vi "Nonfunctional Low rep rate beam pointing correction from kHz images.vi"() -> ()   [LabVIEW 2020]
doc: "The Parallel Processing (Optimized Performance) example shows how to process multiple images in parallel when using a ring acquisition. Images acquired from a camera are stored in a ring buffer and references to each image are pushed to a queue. Each worker loop removes a reference from the queue and processes the image.\n\nIn this example, image processing is simulated by a time delay that can be adjusted while the VI is running. When processing is complete, <B>IMAQdx Release Image</B> must be called in order to free space in the ring buffer."
uses:
  <vilib>/vision/Image Controls.llb/IMAQ Image.ctl
  <vilib>/vision/driver/IMAQdx.llb/IMAQdx Acquisition Mode.ctl
  <vilib>/vision/driver/IMAQdx.llb/IMAQdx Buffer Number Mode.ctl
  <vilib>/vision/driver/NI_Vision_Acquisition_Software.lvlib
  <resource>/objmgr/imaqdx.rc
panel:
  out "remaining elements":T2(array[cluster])
  out "# elements in queue":i32
  out "error out":errorcluster
  out "loop time":u32
  out "Waveform Chart":T3(graph)
  out "Image":T1(plugin-control)
  in  "threshold fraction":sgl=0.8
  in  "Use threshold fraction":bool=TRUE
  out "Images Saved Per Second":dbl
  out "Images Acquired Per Second":dbl
  out "Images Behind":u32
  in  "Range":cluster{"Lower value":sgl, "Upper value":sgl}={"Lower value"=128.0, "Upper value"=255.0} caption="Threshold Range" {"Upper value" format="%.2f"; "Lower value" format="%.2f"}
  out "Lost Buffer Count":u32
  in  "Max # images in memory":i32=200
  out "Images in Queue":i32
  out "Images Processed":u32
  out "Current Buffer Number":u32
  in  "Camera Name":refnum<k21> caption="IMAQdx Session"
  in  "Stop":bool
  # "Overview: Processes multiple extracted images in parallel when using a ring acquisition.\nRequirements: Vision Acquisition Software\nInstructions:\n1. Select the Camera Name\n2. Run the VI"
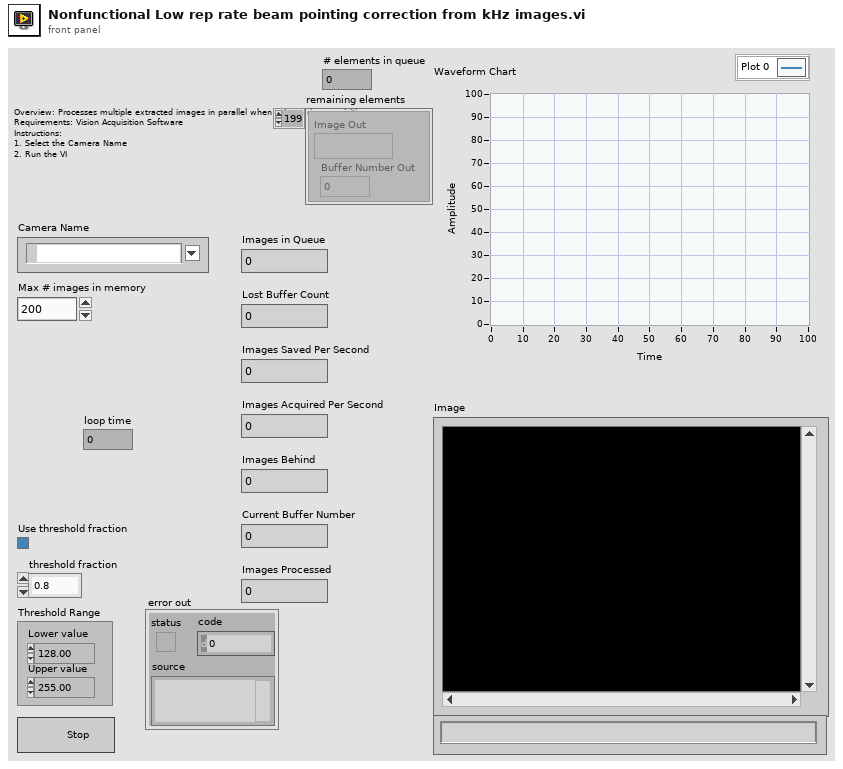
[diagram p1: front panel]
types:
  T1 = typedef "IMAQ Image.ctl" = refnum<image>
  T2 = cluster{"Image Out":T1, "Buffer Number Out":u32}[]
  T3 = cluster{"X Centroid":sgl, "Y Centroid":sgl, "X Centroid":sgl, "Y Centroid":sgl}
  T4 = typedef "IMAQdx.ctl" = refnum<k21>
  T5 = typedef "NI_Vision_Acquisition_Software.lvlib/IMAQdx Acquisition Mode.ctl" = enum32{"One Shot", "Continuous"}
  T6 = typedef "NI_Vision_Acquisition_Software.lvlib/IMAQdx Buffer Number Mode.ctl" = enum32{"Next", "Last", "Buffer Number", "Every", "Last New"}
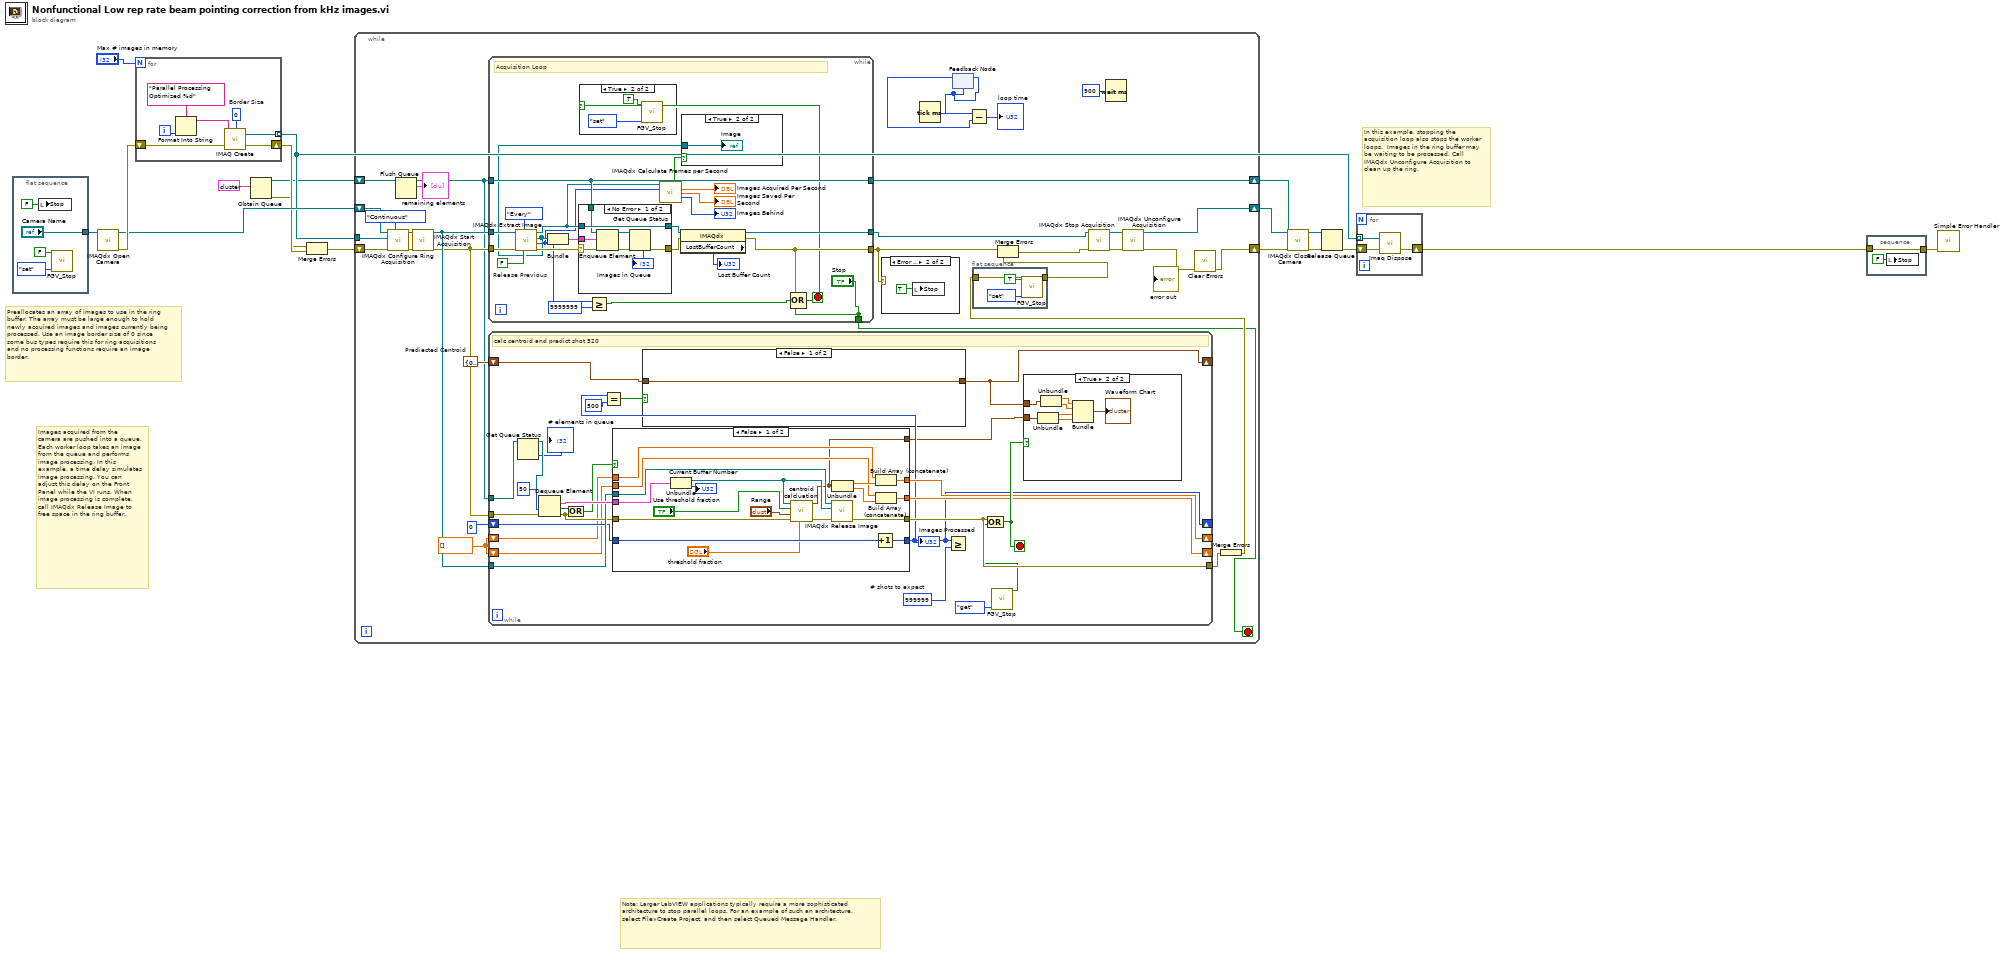
[diagram p0: block diagram]
diagram:
  # "In this example, stopping the acquisition loop also stops the worker loops.  Images in the ring buffer may be waiting to be processed. Call IMAQdx Unconfigure Acquisition to clean up the ring."
  # "Images acquired from the camera are pushed into a queue. Each worker loop takes an image from the queue and performs image processing. In this example, a time delay simulates image processing. You can adjust this delay on the Front Panel while the VI runs. When image processing is complete, call IMAQdx Release Image to free space in the ring buffer."
  # "Preallocates an array of images to use in the ring buffer. The array must be large enough to hold newly acquired images and images currently being processed. Use an image border size of 0 since some bus types require this for ring acquisitions and no processing functions require an image border."
  # "Note: Larger LabVIEW applications typically require a more sophisticated architecture to stop parallel loops. For an example of such an architecture, select File»Create Project, and then select Queued Message Handler."
  n1 = flat-sequence {
    tunnel: ["Camera Name"] -> w15
    frame #0 {
      n2 = local write "Stop"(FALSE ("Stop")) -> ()
      n3 = call "FGV_Stop.vi"("command"=enum16{"set", "get"}."set", "stop"=FALSE) -> ()  [unwired: 9 in, 1 out]
    }
  }
  n4 = call <vilib>:"IMAQdx Open Camera.vi"("Session In"=w15) -> ("error out"=w12:errorcluster, "Session Out"=w11:T4)  [unwired: 2 in, 7 out]
  n5 = for {
    N: "Max # images in memory" -> [_]
    tunnel: [w27] -> w4 mode=indexing
    shift-right: [w26] -> w8
    shift-left: w12 -> [w28]
    i -> [w25]
    w22 = 0  # Border Size
    n6 = Format Into String(format string="Parallel Processing Optimized %d" ("Image Name"), w25) -> (resulting string=w24:string)  [unwired: 2 in, 1 out]
    n7 = call "IMAQ Create"("Border Size"=w22, "Image Name"=w24, "error in (no error)"=w28) -> ("New Image"=w27:T1, "error out"=w26:errorcluster)  [unwired: 1 in, 1 out]
  }
  n8 = Obtain Queue(element data type=cluster{"Image Out":T1, "Buffer Number Out":u32} {"Image Out"=refnum, "Buffer Number Out"=0}) -> (queue out=w1:refnum<queue>, error out=w7:errorcluster)  [unwired: 4 in, 1 out]
  n9 = Merge Errors(w7, w8) -> (w9:errorcluster)
  n10 = while {
    tunnel: w4 -> [w49]
    shift-right: [w59] -> w13
    shift-left: w11 -> [w54]
    shift-right: [w34] -> w14
    shift-left: w9 -> [w52]
    shift-right: [w50] -> w5
    shift-left: w1 -> [w32]
    stop <- w29 stop-if-true
    w39 = cluster{"X Centroid":sgl, "Y Centroid":sgl} {"X Centroid"=0.0, "Y Centroid"=0.0}  # Prediected Centroid
    w40 = sgl[] []
    n11 = call <vilib>:"IMAQdx Configure Ring Acquisition.vi"("Mode"=IMAQdx_Acquisition_Mode."Continuous" ("Continuous?"), "error in"=w52, "Images"=w49, "Session In"=w54) -> ("error out"=w55:errorcluster, "Session Out"=w56:T4)  [unwired: 5 in, 1 out]
    n12 = Flush Queue(queue=w32) -> (queue out=w31:refnum<queue>, remaining elements=→"remaining elements":T2)  [unwired: 1 in, 1 out]
    n13 = call <vilib>:"IMAQdx Start Acquisition.vi"("error in"=w55, "Session In"=w56) -> ("error out"=w46:errorcluster, "Session Out"=w47:T4)  [unwired: 8 out]
    n14 = while {
      tunnel: w46 -> [w144]
      tunnel: w47 -> [w141]
      tunnel: w31 -> [w134]
      tunnel: [w140] -> w48
      tunnel: [w138] -> w45
      tunnel: [w134] -> w50
      tunnel: ["Stop"] -> w29
      stop <- w122 stop-if-true
      w142 = FALSE  # Release Previous
      # "Acquisition Loop"
      n15 = call <vilib>:"IMAQdx Extract Image.vi"("Release Previous (true)"=w142, "Buffer Number Mode (Next)"=IMAQdx_Buffer_Number_Mode."Every" ("Buffer Number Mode"), "error in"=w144, "Session In"=w141) -> ("error out"=w137:errorcluster, "Buffer Number Out"=w125:u32, "Image Out"=w127:T1, "Session Out"=w129:T4)  [unwired: 4 in]
      n16 = Bundle("Image Out"=w127, "Buffer Number Out"=w125) -> (w135:cluster{"Image Out":T1, "Buffer Number Out":u32})  [unwired: 1 in]
      n17 = case shown="No Error" w137 {
        selector: w137 -> [w151 w156]
        tunnel: [w152 w157] -> w136
        tunnel: w129 -> [w152 w157]
        tunnel: w135 -> [w150 _]
        tunnel: w134 -> [w149 _]
        tunnel: [w148 w156] -> w133
        frame No Error {
          n18 = Enqueue Element(queue=w149, element=w150, error in (no error)=w151) -> (queue out=w154:refnum<queue>, error out=w155:errorcluster)  [unwired: 1 in, 1 out]
          n19 = Get Queue Status(queue=w154, error in (no error)=w155) -> (error out=w148:errorcluster, # elements in queue=→"Images in Queue":i32)  [unwired: 1 in, 6 out]
        }
        frame Error {
        }
      }
      n20 = Greater Or Equal?(x=w125, y=u32 9999999) -> (x >= y?=w123:bool)
      n21 = call <vilib>:"IMAQdx Calculate Frames per Second.vi"("Session In"=w129, "Buffer Number"=w125) -> ("Update Display"=w128:bool, "Acquired Frames per Second"=→"Images Acquired Per Second":dbl, "Processed Frames per Second"=→"Images Saved Per Second":dbl, "Images Behind"=→"Images Behind":i32)  [unwired: 7 in, 3 out]
      n22 = property class="IMAQdx"(reference=w136, error in=w133) -> (reference out=w140:T4, error out=w138:errorcluster, "LostBufferCount"=→"Lost Buffer Count":u32)
      n23 = case shown="True" w128 {
        tunnel: w127 -> [_ w147]
        frame False {
        }
        frame True {
          "Image" <- w147
        }
      }
      n24 = Compound Arithmetic op=OR(w138, w123, "Stop") -> (w122:bool)
      n25 = case shown="True" w122 {
        frame False {
        }
        frame True {
          n26 = call "FGV_Stop.vi"("command"=enum16{"set", "get"}."set", "stop"=TRUE) -> ()  [unwired: 9 in, 1 out]
        }
      }
    }
    n27 = while {
      tunnel: [w75] -> w41
      tunnel: w31 -> [w64]
      tunnel: w47 -> [w83]
      shift-right: [w68] -> _
      shift-left: u32 0 -> [w82]
      tunnel: w46 -> [w81]
      shift-right: [w73] -> _
      shift-left: w40 -> [w74]
      shift-right: [w72] -> _
      shift-left: w40 -> [w71]
      shift-right: [w66] -> _
      shift-left: w39 -> [w67]
      stop <- w76 stop-if-true
      w77 = i64 999999  # # shots to expect
      # "calc centroid and predict shot 520"
      n28 = Get Queue Status(queue=w64) -> (queue out=w63:refnum<queue>, # elements in queue=→"# elements in queue":i32)  [unwired: 2 in, 6 out]
      n29 = Dequeue Element(queue=w63, timeout in ms (-1)=50 ("timeout in ms"), error in (no error)=w81) -> (element=w84:cluster{"Image Out":T1, "Buffer Number Out":u32}, timed out?=w79:bool, error out=w78:errorcluster)  [unwired: 1 out]
      n30 = Or(x=w79, y=w78) -> (x .or. y?=w80:bool)
      n31 = case shown="False" w80 {
        tunnel: w78 -> [w107 w117]
        tunnel: w84 -> [w113 _]
        tunnel: [w112 w117] -> w75
        tunnel: w83 -> [w111 _]
        tunnel: w82 -> [w109 w116]
        tunnel: [w108 w116] -> w68
        tunnel: w74 -> [w101 w115]
        tunnel: [w99 w115] -> w73
        tunnel: [w97 w114] -> w72
        tunnel: w71 -> [w96 w114]
        tunnel: [w95 _] -> w65
        frame False {
          n32 = Unbundle(w113) -> ("Image Out"=w104:T1, "Buffer Number Out"=→"Current Buffer Number":u32)
          n33 = call "centroid calcluation.vi"("threshold fraction"="threshold fraction", "error in (no error)"=w107, "Range"="Range", "Use threshold fraction"="Use threshold fraction", "Refnum in"=w104) -> ("error out"=w106:errorcluster, "Centroid"=w95:cluster{"X Centroid":sgl, "Y Centroid":sgl})  [unwired: 4 in, 1 out]
          n34 = call <vilib>:"IMAQdx Release Image.vi"("error in"=w106, "Image"=w104, "Session In"=w111) -> ("error out"=w112:errorcluster)  [unwired: 7 in, 1 out]
          n35 = Unbundle(w95) -> ("X Centroid"=w100:sgl, "Y Centroid"=w98:sgl)
          n36 = Increment(x=w109) -> (x+1=w108:u32)
          n37 = Build Array (concatenate)(w101, w100) -> (w99:sgl[])
          n38 = Build Array (concatenate)(w96, w98) -> (w97:sgl[])
        }
        frame True {
          # "Empty queue or error.\nNothing to process."
        }
      }
      "Images Processed" <- w68
      n39 = Equal?(x=w68, y=u32 500) -> (x = y?=w69:bool)
      n40 = case shown="False" w69 {
        tunnel: w67 -> [w86 w87]
        tunnel: [w86 w87] -> w66
        frame False {
        }
        frame True {
          # "send to Python. Get predicted centroid"
        }
      }
      n41 = Greater Or Equal?(x=w68, y=w77) -> ()  [unwired: 1 out]
      n42 = call "FGV_Stop.vi"("command"=enum16{"set", "get"}."get") -> ("stop"=w60:bool)  [unwired: 10 in]
      n43 = Compound Arithmetic op=OR(w75, w60) -> (w76:bool)
      n44 = case shown="True" w76 {
        tunnel: w66 -> [_ w93]
        tunnel: w65 -> [_ w94]
        frame False {
        }
        frame True {
          n45 = Unbundle(w94) -> ("X Centroid"=w90:sgl, "Y Centroid"=w89:sgl)
          n46 = Unbundle(w93) -> ("X Centroid"=w92:sgl, "Y Centroid"=w91:sgl)
          n47 = Bundle("X Centroid"=w92, "Y Centroid"=w91, "X Centroid"=w90, "Y Centroid"=w89) -> (→"Waveform Chart":T3)  [unwired: 1 in]
        }
      }
    }
    n48 = case shown="Error .." w45 {
      frame No Error {
      }
      frame Error {
        n49 = local write "Stop"(TRUE ("Stop")) -> ()
      }
    }
    n50 = Tick Count (ms)() -> (millisecond timer value=w38:u32)
    n51 = feedback #1(w38) -> (w37:u32)
    n52 = feedback-in #1(w38) -> ()
    n53 = Subtract(x=w38, y=w37) -> (x-y=→"loop time":u32)
    n54 = flat-sequence {
      tunnel: w44 -> [w118]
      tunnel: [w118] -> w43
      frame #0 {
        n55 = call "FGV_Stop.vi"("command"=enum16{"set", "get"}."set", "stop"=TRUE) -> ()  [unwired: 9 in, 1 out]
      }
    }
    n56 = Merge Errors(w45, w43) -> (w51:errorcluster)
    n57 = call <vilib>:"IMAQdx Stop Acquisition.vi"("error in"=w51, "Session In"=w48) -> ("error out"=w57:errorcluster, "Session Out"=w58:T4)  [unwired: 8 out]
    n58 = Wait (ms)(milliseconds to wait=u32 900) -> ()  [unwired: 1 out]
    n59 = call <vilib>:"IMAQdx Unconfigure Acquisition.vi"("error in"=w57, "Session In"=w58) -> ("error out"=w35:errorcluster, "Session Out"=w59:T4)  [unwired: 8 out]
    "error out" <- w35
    n60 = call <vilib>:"Clear Errors.vi"("error in (no error)"=w35) -> ("error out"=w34:errorcluster)  [unwired: 5 in, 1 out]
    n61 = Merge Errors(w41) -> (w44:errorcluster)
  }
  n62 = call <vilib>:"IMAQdx Close Camera.vi"("error in"=w14, "Session In"=w13) -> ("error out"=w3:errorcluster)  [unwired: 9 out]
  n63 = Release Queue(queue=w5, error in (no error)=w3) -> (error out=w2:errorcluster)  [unwired: 1 in, 2 out]
  n64 = for {
    shift-right: [w159] -> w16
    shift-left: w2 -> [w160]
    tunnel: w4 -> [w158] mode=indexing
    n65 = call "Imaq Dispose"("Image"=w158, "error in (no error)"=w160) -> ("error out"=w159:errorcluster)  [unwired: 4 in]
  }
  n66 = stacked-sequence {
    tunnel: [w161] -> w17
    tunnel: w16 -> [w161]
    frame #0 {
      n67 = local write "Stop"(FALSE ("Stop")) -> ()
    }
  }
  n68 = call <vilib>:"Simple Error Handler.vi"("error in (no error)"=w17) -> ()  [unwired: 4 in, 5 out]
